vi "Get Object Entry.vi"(8 "error in":errorcluster, 10 "OD Index":u16 format="%.0x", 11 "Obj Dict in":refnum<class "Object Dictionary.lvclass">) -> (0 "error out":errorcluster, 1 "Obj Entry":refnum<class "Object Entry.lvclass">, 3 "Obj Dict out":refnum<class "Object Dictionary.lvclass">)   [LabVIEW 2020, in "CANopen.lvlib" / "Object Dictionary.lvclass"]
uses:
  Object Dictionary.lvclass
  Object Entry/Object Entry.lvclass
  Object Dictionary.lvclass/Object Dictionary.ctl
  Ordered-Dictionary/Ordered Object Dictionary/Source/Ordered Object Dictionary.lvclass
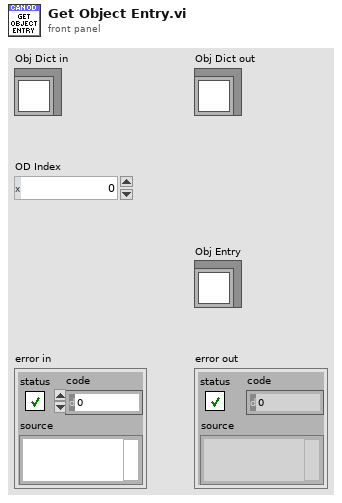
[diagram p1: front panel]
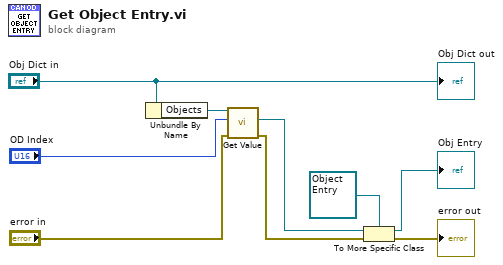
[diagram p0: block diagram]
diagram:
  n1 = Unbundle By Name("Obj Dict in") -> ("Objects"=w8:refnum<class "Ordered Object Dictionary.lvclass">)
  n2 = call "Get Value.vi"("error in"="error in", "Key"="OD Index", "Ordered Object Dictionary in"=w8) -> ("error out"=w5:errorcluster, "Value"=w3:refnum<class>)  [unwired: 6 in, 1 out]
  n3 = To More Specific Class(target class=refnum<class "Object Entry.lvclass"> refnum ("CANopen Object Dictionary.lvlib:Obj Entry"), reference=w3, error in=w5) -> (specific class reference=→"Obj Entry":refnum<class "Object Entry.lvclass">, error out=→"error out":errorcluster)
  "Obj Dict out" <- "Obj Dict in"
